vi "FileParse.vi"(10 "all rows":dbl[][](array[numeric])) -> ()   [LabVIEW 2014]
uses:
  Common Code/commandCluster.ctl
  Robot Global Data.vi
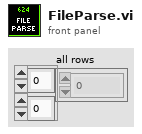
[diagram p1: front panel]
types:
  T1 = typedef "commandCluster.ctl" = cluster{"Step ID":i16, "Command Type":i16, "Drive X":sgl, "Drive Y":sgl, "Heading":sgl, "Max Exec. Time":i16, "Jump Type":i32, "Jump To":i16, "Jump Condition":i16, "Async Drive?":i16, "Roller Mode":i16, "Roller Align":i16, "Roller Closed?":i16, "Wait Condition":i16, "Elevator Mode":i16, "Elevator Command":i16, "Roller State":i16, "Hold Low?":i16, "Num Totes":i16, "Num Cans":dbl, "Past Distance":dbl, "Store Can?":dbl, "X Speed":dbl, "Y Speed":dbl, "Yaw Angle Set":dbl, "Grab Can":dbl, "Roller Overide Speed":dbl, "Force Load?":sgl, "Set Idle":sgl, "Eject":sgl, "Pike Action":sgl, "Pivot Speed":dbl, "Height":dbl}
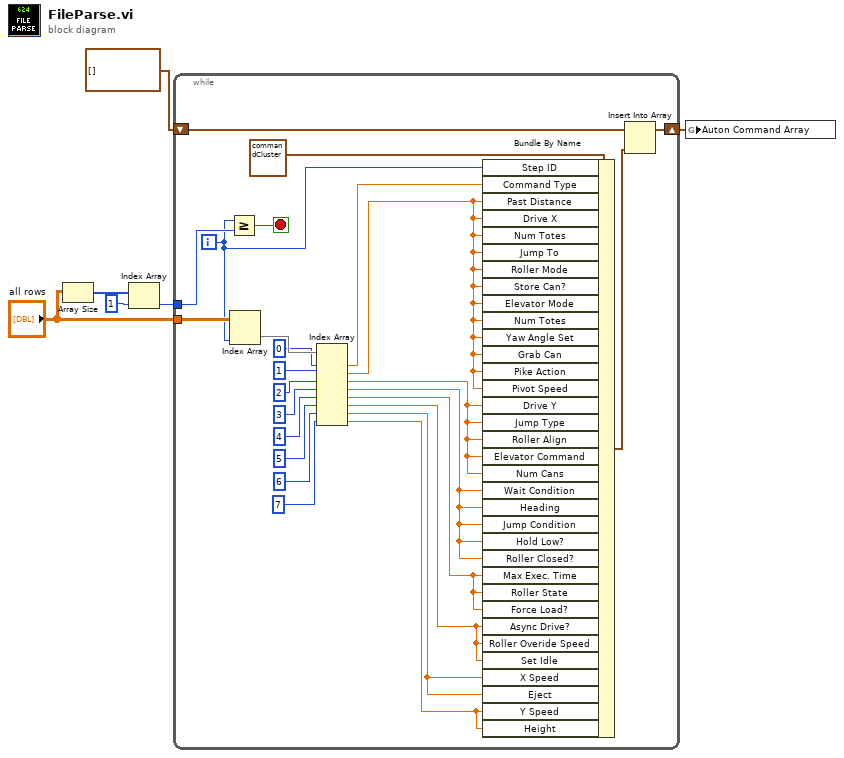
[diagram p0: block diagram]
diagram:
  n1 = Array Size(array="all rows") -> (size(s)=w6:i32[])
  n2 = Index Array(array=w6, index=1) -> (element=w4:i32)
  n3 = while {
    tunnel: w4 -> [w31]
    tunnel: "all rows" -> [w29]
    shift-right: [w20] -> w1
    shift-left: T1[] [] -> [w19]
    i -> [w18]
    stop <- w30 stop-if-true
    n4 = Greater Or Equal?(x=w18, y=w31) -> (x >= y?=w30:bool)
    n5 = Index Array(array=w29, index (col)=w18) -> (element=w28:dbl[])  [unwired: 1 in]
    n6 = Index Array(array=w28, index #1=0 ("index"), index #2=1 ("index"), index #3=2 ("index"), index #4=3 ("index"), index #5=4 ("index"), index #6=5 ("index"), index #7=6 ("index"), index #8=7 ("index")) -> (element #1=w17:dbl, element #2=w8:dbl, element #3=w16:dbl, element #4=w15:dbl, element #5=w11:dbl, element #6=w10:dbl, element #7=w9:dbl, element #8=w7:dbl)
    n7 = Bundle By Name(cluster=T1 {"Step ID"=0, "Command Type"=0, "Drive X"=0.0, "Drive Y"=0.0, "Heading"=0.0, "Max Exec. Time"=0, "Jump Type"=0, "Jump To"=0, "Jump Condition"=0, "Async Drive?"=0, "Roller Mode"=0, "Roller Align"=0, "Roller Closed?"=0, "Wait Condition"=0, "Elevator Mode"=0, "Elevator Command"=0, "Roller State"=0, "Hold Low?"=0, "Num Totes"=0, "Num Cans"=0.0, "Past Distance"=0.0, "Store Can?"=0.0, "X Speed"=0.0, "Y Speed"=0.0, "Yaw Angle Set"=0.0, "Grab Can"=0.0, "Roller Overide Speed"=0.0, "Force Load?"=0.0, "Set Idle"=0.0, "Eject"=0.0, "Pike Action"=0.0, "Pivot Speed"=0.0, "Height"=0.0} ("Command Cluster"), "Step ID"=w18, "Command Type"=w17, "Past Distance"=w8, "Drive X"=w8, "Num Totes"=w8, "Jump To"=w8, "Roller Mode"=w8, "Store Can?"=w8, "Elevator Mode"=w8, "Num Totes"=w8, "Yaw Angle Set"=w8, "Grab Can"=w8, "Pike Action"=w8, "Pivot Speed"=w8, "Drive Y"=w16, "Jump Type"=w16, "Roller Align"=w16, "Elevator Command"=w16, "Num Cans"=w16, "Wait Condition"=w15, "Heading"=w15, "Jump Condition"=w15, "Hold Low?"=w15, "Roller Closed?"=w15, "Max Exec. Time"=w11, "Roller State"=w11, "Force Load?"=w11, "Async Drive?"=w10, "Roller Overide Speed"=w10, "Set Idle"=w10, "X Speed"=w9, "Eject"=w9, "Y Speed"=w7, "Height"=w7) -> (w27:T1)
    n8 = Insert Into Array(array=w19, new element=w27) -> (w20:T1[])  [unwired: 1 in]
  }
  n9 = global write "Robot Global Data.vi" "Auton Command Array"(w1) -> ()
